vi "VisionDashRead_LeftFront.vi"(8 "error in (no error)":errorcluster) -> (0 "error out":errorcluster)   [LabVIEW 2023]
doc: "Vision Network\n\nInput\n --Error in \n\nOutput\n --Error out"
uses:
  VisionGlobal.vi
  <vilib>/Rock Robotics/Network Tables/NT Write Integer.vi
  <vilib>/Rock Robotics/Network Tables/NT Write Boolean.vi
  <vilib>/Rock Robotics/Network Tables/NT Write Number.vi
  <vilib>/Rock Robotics/WPI/ThirdParty/JAS_Junk/TrajLib/Trajectory_Library.lvlib
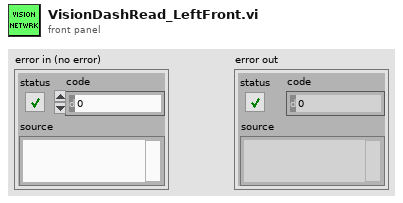
[diagram p1: front panel]
types:
  T1 = typedef "Trajectory_Library.lvlib/POSE2D.ctl" = cluster{"TRANSLATION":T2, "ROTATION":T3}
  T2 = typedef "Trajectory_Library.lvlib/TRANSLATION2D.ctl" = cluster{"X":dbl, "Y":dbl}
  T3 = typedef "Trajectory_Library.lvlib/ROTATION2D.ctl" = cluster{"VALUE":dbl, "COS":dbl, "SIN":dbl}
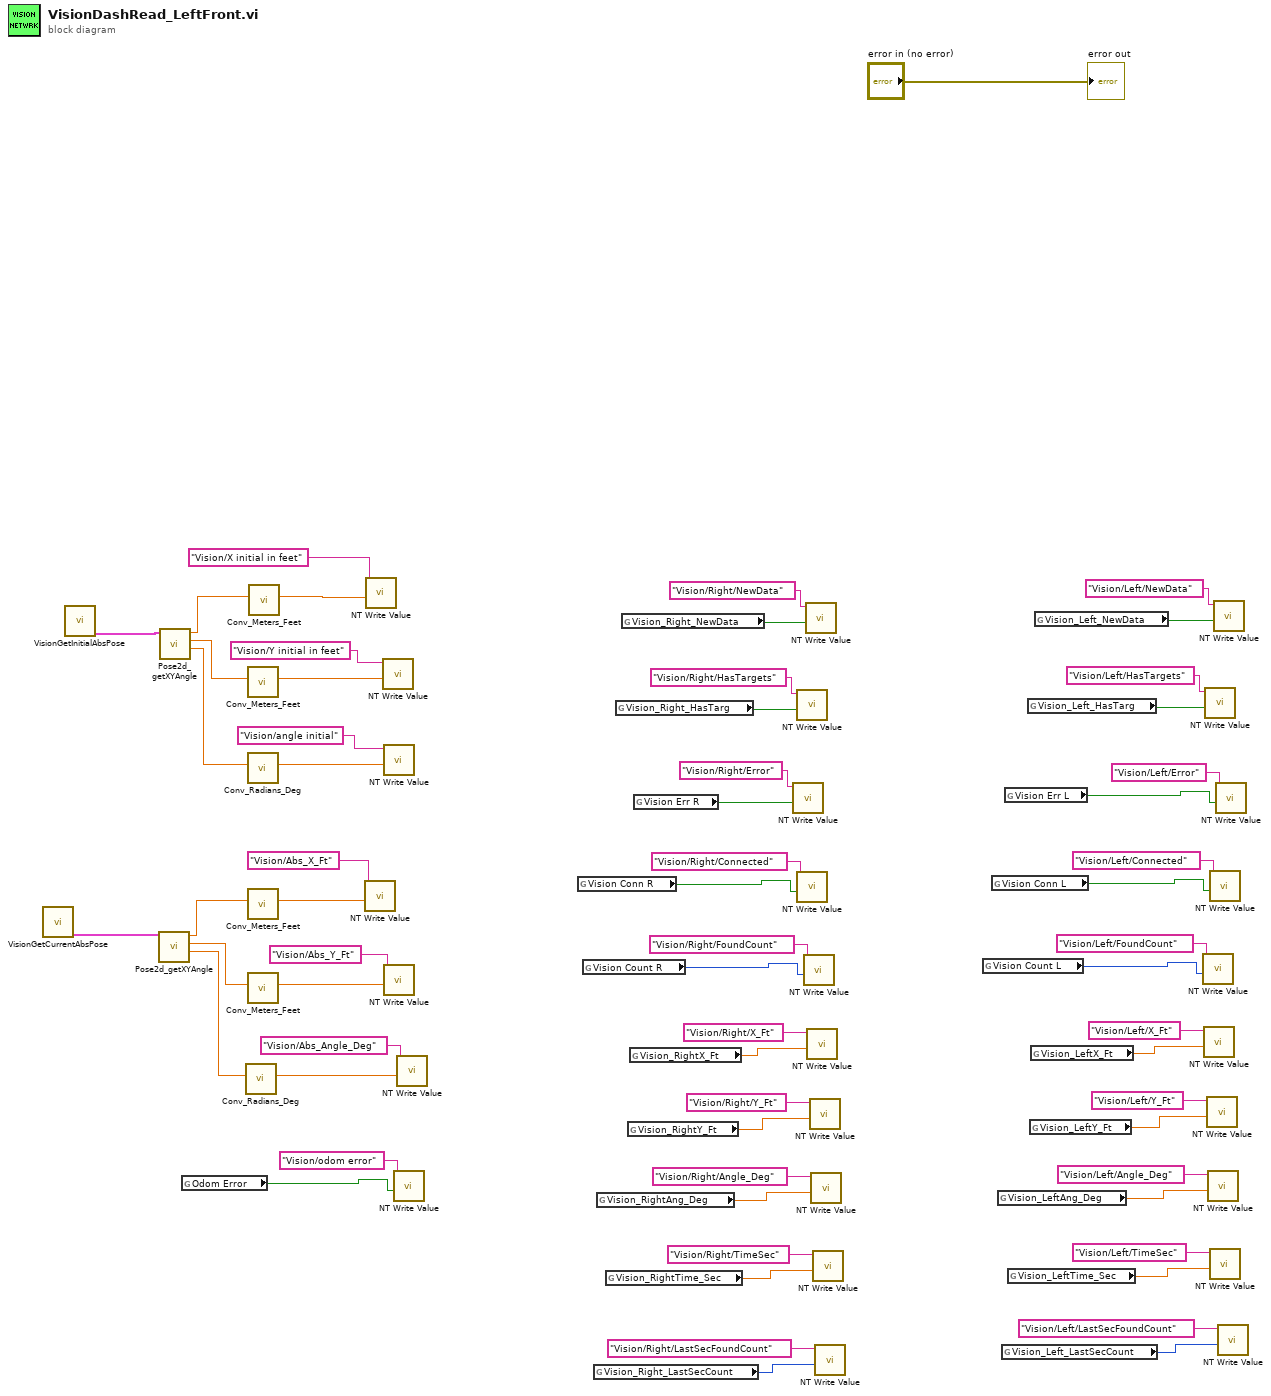
[diagram p0: block diagram]
diagram:
  n1 = call "VisionGetCurrentAbsPose.vi"() -> ("Current ABS Pose"=w62:T1)  [unwired: 9 in]
  n2 = call "VisionGetInitialAbsPose.vi"() -> ("InitialABSPose"=w49:T1)  [unwired: 10 in]
  n3 = call <vilib>:"Pose2d_getXYAngle.vi"("in POSE"=w62) -> ("Angle"=w61:dbl, "Y"=w60:dbl, "X"=w59:dbl)  [unwired: 8 in]
  n4 = call <vilib>:"Pose2d_getXYAngle.vi"("in POSE"=w49) -> ("Angle"=w55:dbl, "Y"=w54:dbl, "X"=w53:dbl)  [unwired: 8 in]
  n5 = global read "VisionGlobal.vi" "Odom Error"() -> (w41:bool)
  n6 = call <vilib>:"Conv_Radians_Deg.vi"("Radians"=w61) -> ("Degrees"=w56:dbl)  [unwired: 10 in]
  n7 = call <vilib>:"Conv_Meters_Feet.vi"("Meters"=w54) -> ("Feet"=w51:dbl)  [unwired: 10 in]
  n8 = call <vilib>:"Conv_Radians_Deg.vi"("Radians"=w55) -> ("Degrees"=w50:dbl)  [unwired: 10 in]
  n9 = call <vilib>:"Conv_Meters_Feet.vi"("Meters"=w59) -> ("Feet"=w58:dbl)  [unwired: 10 in]
  n10 = call <vilib>:"Conv_Meters_Feet.vi"("Meters"=w60) -> ("Feet"=w57:dbl)  [unwired: 10 in]
  n11 = call <vilib>:"Conv_Meters_Feet.vi"("Meters"=w53) -> ("Feet"=w52:dbl)  [unwired: 10 in]
  n12 = call-poly <vilib>:"NT Write Value.vi"("value"=w58, "name"="Vision/Abs_X_Ft") -> ()  [unwired: 9 in, 1 out]
  n13 = call-poly <vilib>:"NT Write Value.vi"("value"=w52, "name"="Vision/X initial in feet") -> ()  [unwired: 9 in, 1 out]
  n14 = call-poly <vilib>:"NT Write Value.vi"("value"=w51, "name"="Vision/Y initial in feet") -> ()  [unwired: 9 in, 1 out]
  n15 = call-poly <vilib>:"NT Write Value.vi"("value"=w50, "name"="Vision/angle initial") -> ()  [unwired: 9 in, 1 out]
  n16 = call-poly <vilib>:"NT Write Value.vi"("value"=w57, "name"="Vision/Abs_Y_Ft") -> ()  [unwired: 9 in, 1 out]
  n17 = call-poly <vilib>:"NT Write Value.vi"("value"=w41, "name"="Vision/odom error") -> ()  [unwired: 9 in, 1 out]
  n18 = call-poly <vilib>:"NT Write Value.vi"("value"=w56, "name"="Vision/Abs_Angle_Deg") -> ()  [unwired: 9 in, 1 out]
  n19 = global read "VisionGlobal.vi" "Vision Conn R"() -> (w32:bool)
  n20 = global read "VisionGlobal.vi" "Vision Count R"() -> (w30:i32)
  n21 = global read "VisionGlobal.vi" "Vision_Right_LastSecCount"() -> (w3:i32)
  n22 = global read "VisionGlobal.vi" "Vision_RightAng_Deg"() -> (w21:dbl)
  n23 = global read "VisionGlobal.vi" "Vision_RightTime_Sec"() -> (w24:dbl)
  n24 = global read "VisionGlobal.vi" "Vision_Right_HasTarg"() -> (w12:bool)
  n25 = global read "VisionGlobal.vi" "Vision_Right_NewData"() -> (w10:bool)
  n26 = global read "VisionGlobal.vi" "Vision_RightY_Ft"() -> (w22:dbl)
  n27 = global read "VisionGlobal.vi" "Vision_RightX_Ft"() -> (w23:dbl)
  n28 = global read "VisionGlobal.vi" "Vision Err R"() -> (w34:bool)
  n29 = call-poly <vilib>:"NT Write Value.vi"("value"=w34, "name"="Vision/Right/Error") -> ()  [unwired: 9 in, 1 out]
  n30 = call-poly <vilib>:"NT Write Value.vi"("value"=w12, "name"="Vision/Right/HasTargets") -> ()  [unwired: 9 in, 1 out]
  n31 = call-poly <vilib>:"NT Write Value.vi"("value"=w32, "name"="Vision/Right/Connected") -> ()  [unwired: 9 in, 1 out]
  n32 = call-poly <vilib>:"NT Write Value.vi"("value"=w30, "name"="Vision/Right/FoundCount") -> ()  [unwired: 9 in, 1 out]
  n33 = call-poly <vilib>:"NT Write Value.vi"("value"=w10, "name"="Vision/Right/NewData") -> ()  [unwired: 9 in, 1 out]
  n34 = call-poly <vilib>:"NT Write Value.vi"("value"=w23, "name"="Vision/Right/X_Ft") -> ()  [unwired: 9 in, 1 out]
  n35 = call-poly <vilib>:"NT Write Value.vi"("value"=w22, "name"="Vision/Right/Y_Ft") -> ()  [unwired: 9 in, 1 out]
  n36 = call-poly <vilib>:"NT Write Value.vi"("value"=w21, "name"="Vision/Right/Angle_Deg") -> ()  [unwired: 9 in, 1 out]
  n37 = call-poly <vilib>:"NT Write Value.vi"("value"=w24, "name"="Vision/Right/TimeSec") -> ()  [unwired: 9 in, 1 out]
  n38 = call-poly <vilib>:"NT Write Value.vi"("value"=w3, "name"="Vision/Right/LastSecFoundCount") -> ()  [unwired: 9 in, 1 out]
  n39 = global read "VisionGlobal.vi" "Vision Count L"() -> (w39:i32)
  n40 = global read "VisionGlobal.vi" "Vision Conn L"() -> (w35:bool)
  n41 = global read "VisionGlobal.vi" "Vision_LeftAng_Deg"() -> (w13:dbl)
  n42 = global read "VisionGlobal.vi" "Vision_Left_LastSecCount"() -> (w1:i32)
  n43 = global read "VisionGlobal.vi" "Vision Err L"() -> (w37:bool)
  n44 = global read "VisionGlobal.vi" "Vision_LeftTime_Sec"() -> (w16:dbl)
  n45 = global read "VisionGlobal.vi" "Vision_Left_HasTarg"() -> (w8:bool)
  n46 = global read "VisionGlobal.vi" "Vision_LeftY_Ft"() -> (w14:dbl)
  n47 = global read "VisionGlobal.vi" "Vision_LeftX_Ft"() -> (w15:dbl)
  n48 = global read "VisionGlobal.vi" "Vision_Left_NewData"() -> (w6:bool)
  n49 = call-poly <vilib>:"NT Write Value.vi"("value"=w39, "name"="Vision/Left/FoundCount") -> ()  [unwired: 9 in, 1 out]
  n50 = call-poly <vilib>:"NT Write Value.vi"("value"=w15, "name"="Vision/Left/X_Ft") -> ()  [unwired: 9 in, 1 out]
  n51 = call-poly <vilib>:"NT Write Value.vi"("value"=w8, "name"="Vision/Left/HasTargets") -> ()  [unwired: 9 in, 1 out]
  n52 = call-poly <vilib>:"NT Write Value.vi"("value"=w14, "name"="Vision/Left/Y_Ft") -> ()  [unwired: 9 in, 1 out]
  n53 = call-poly <vilib>:"NT Write Value.vi"("value"=w13, "name"="Vision/Left/Angle_Deg") -> ()  [unwired: 9 in, 1 out]
  n54 = call-poly <vilib>:"NT Write Value.vi"("value"=w35, "name"="Vision/Left/Connected") -> ()  [unwired: 9 in, 1 out]
  n55 = call-poly <vilib>:"NT Write Value.vi"("value"=w16, "name"="Vision/Left/TimeSec") -> ()  [unwired: 9 in, 1 out]
  n56 = call-poly <vilib>:"NT Write Value.vi"("value"=w6, "name"="Vision/Left/NewData") -> ()  [unwired: 9 in, 1 out]
  n57 = call-poly <vilib>:"NT Write Value.vi"("value"=w37, "name"="Vision/Left/Error") -> ()  [unwired: 9 in, 1 out]
  n58 = call-poly <vilib>:"NT Write Value.vi"("value"=w1, "name"="Vision/Left/LastSecFoundCount") -> ()  [unwired: 9 in, 1 out]
  "error out" <- "error in (no error)"
